vi "PR Set No Acq Signal.vi"(1 "Number":i32) -> (0 "NoAcqSignal":i32)   [LabVIEW 2022 SP3, in "BS6006PRPLUS.lvlib"]
doc: "The function sets the number of signals to be acquired. The product of Number and Length, which is the input parameter of PR_SetLengthOfSignal, should be less than 262144.\n\nextern \"C\" BS6006PRPLUS_API int __cdecl PR_SetNoAcqSignal(int Number);"
uses:
  BS6006PRPLUS.lvlib
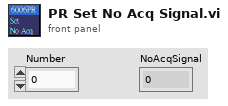
[diagram p1: front panel]
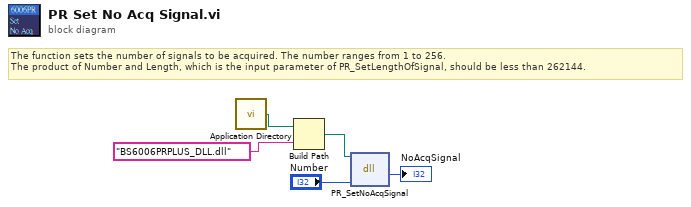
[diagram p0: block diagram]
diagram:
  # "The function sets the number of signals to be acquired. The number ranges from 1 to 256.\nThe product of Number and Length, which is the input parameter of PR_SetLengthOfSignal, should be less than 262144."
  n1 = call <vilib>:"Application Directory.vi"() -> ("Application Directory"=w3:path)
  n2 = Build Path(base path=w3, name or relative path="BS6006PRPLUS_DLL.dll") -> (appended path=w1:path)
  n3 = dll-call lib="E:/Broadsound_Program/PulserReceiver/6006PR PLUS/API/DLL/LabVIEW 15/VIs/BS6006PRPLUS_DLL.dlls" fn="PR_SetNoAcqSignal"(path in=w1, "Number"="Number") -> ("return type"=→"NoAcqSignal":i32)  [unwired: 3 in, 2 out]
